vi "Contro_ERD_Loop.vi"(0 "ERD Loop":refnum<queue>, 11 "Error In":errorcluster, 13 "Command (ERD Loop Control)":T1) -> (15 "Error Out":errorcluster)   [LabVIEW 2021]
uses:
  Controles/Main_Machine_State.ctl
  Controles/Command(ERD Loop Control).ctl
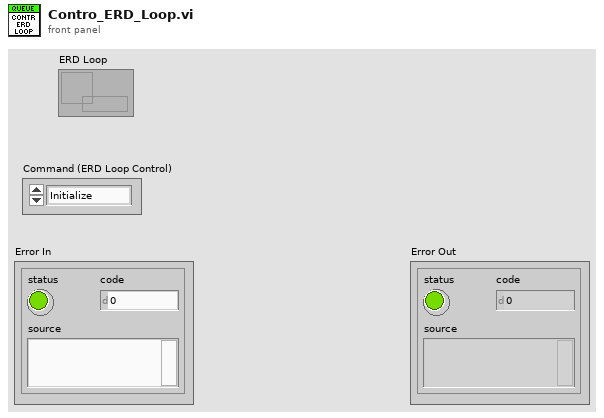
[diagram p1: front panel]
types:
  T1 = typedef "Command(ERD Loop Control).ctl" = enum16{"Initialize", "Shutdown"}
  T2 = typedef "Main_Machine_State.ctl" = enum16{"Init", "Get Version", "Build ERD Read List", "Update UI", "Read ERDs", "Log Data", "Pause", "Shutdown"}
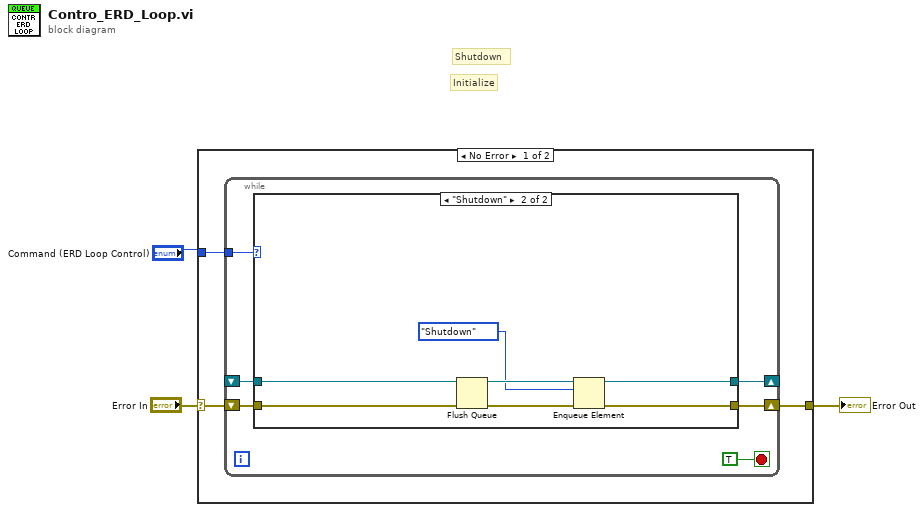
[diagram p0: block diagram]
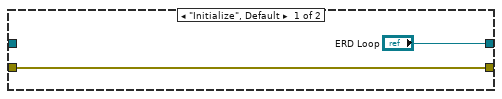
[diagram p2: hidden frame]
diagram:
  # "Initialize"
  # "Shutdown"
  n1 = case shown="No Error" "Error In" {
    selector: "Error In" -> [w5 w22]
    tunnel: "Command (ERD Loop Control)" -> [w6 _]
    tunnel: [w4 w22] -> w2
    frame No Error {
      n2 = while {
        tunnel: w6 -> [w12]
        shift-right: [w9] -> w4
        shift-left: w5 -> [w10]
        shift-right: [w8] -> _
        shift-left: _ -> [w7]
        stop <- TRUE stop-if-true
        n3 = case shown="\"Shutdown\"" w12 {
          tunnel: w10 -> [w14 w21]
          tunnel: [w14 w19] -> w9
          tunnel: ["ERD Loop" w18] -> w8
          tunnel: w7 -> [_ w16]
          frame "Initialize", Default {
          }
          frame "Shutdown" {
            n4 = Flush Queue(queue=w16, error in (no error)=w21) -> (queue out=w17:refnum<queue>, error out=w20:errorcluster)  [unwired: 1 out]
            n5 = Enqueue Element(queue=w17, element=Main_Machine_State."Shutdown", error in (no error)=w20) -> (queue out=w18:refnum<queue>, error out=w19:errorcluster)  [unwired: 1 in, 1 out]
          }
        }
      }
    }
    frame Error {
    }
  }
  "Error Out" <- w2
